vi "getobjlist.vi"(0 "connection":T1, 1 "error in":errorcluster) -> (2 "StringsAndValues[]":cluster{"String":string, "Value":u16}[](array[cluster]), 3 "connection out":T1, 4 "error out":errorcluster)   [LabVIEW 2010]
uses:
  <vilib>/addons/database/Connection.llb/Conn ObjectReference.ctl
  <vilib>/addons/database/NI_Database_API.lvlib
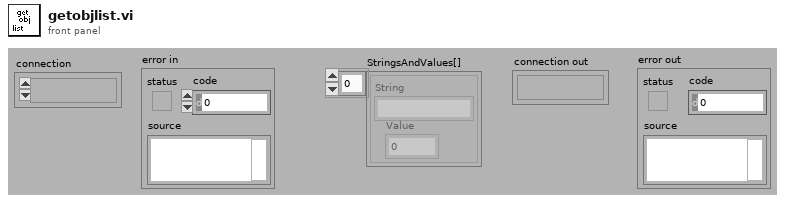
[diagram p1: front panel]
types:
  T1 = typedef "NI_Database_API.lvlib/Conn ObjectReference.ctl" = refnum<k1>
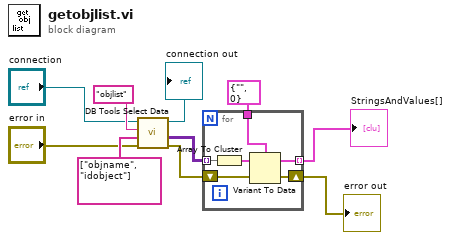
[diagram p0: block diagram]
diagram:
  n1 = call <vilib>:"DB Tools Select Data.vi"("error in (no error)"="error in", "columns"=string[] ["objname", "idobject"], "table"="objlist", "connection reference"="connection") -> ("error out"=w5:errorcluster, "data"=w6:variant[][], "connection reference out"=→"connection out":T1)  [unwired: 2 in]
  n2 = for {
    tunnel: cluster{"String":string, "Value":u16} {"String"="", "Value"=0} -> [w14]
    tunnel: w6 -> [w16] mode=indexing
    tunnel: [w13] -> w7 mode=indexing
    shift-right: [w11] -> w10
    shift-left: w5 -> [w12]
    n3 = Array To Cluster(array=w16) -> (cluster=w15:cluster{"data[0]":variant, "data[1]":variant})
    n4 = Variant To Data(error in=w12, Variant=w15, type=w14) -> (error out=w11:errorcluster, data=w13:cluster{"String":string, "Value":u16})
  }
  "error out" <- w10
  "StringsAndValues[]" <- w7
